vi "Load Words.vi"() -> (3 "Words":string[](array[string]))   [LabVIEW 2020]
uses:
  e4af47f0-1ddf-409f-991e-327bca181c6e.vi
  c56a025f-5e1b-4844-8108-8c9a202df3bb.vi
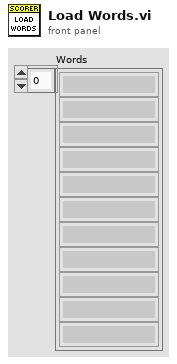
[diagram p1: front panel]
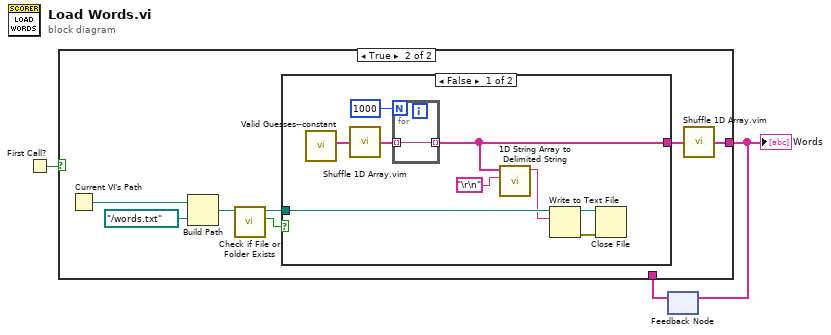
[diagram p0: block diagram]
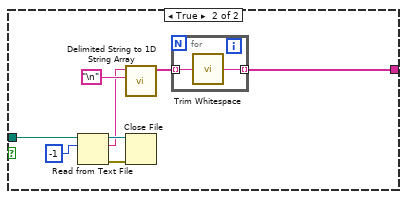
[diagram p3: hidden frame]
diagram:
  n1 = First Call?() -> (First Call?: T/F=w3:bool)
  n2 = feedback #1() -> (w2:string[])  [unwired: 1 in]
  n3 = case shown="True" w3 {
    tunnel: [w4 w6] -> w1
    tunnel: w2 -> [w4 _]
    frame False {
    }
    frame True {
      n4 = Current VI's Path() -> (path=w5:path)
      n5 = Build Path(base path=w5, name or relative path=path "../words.txt") -> (appended path=w10:path)
      n6 = call <vilib>:"Check if File or Folder Exists.vi"("path"=w10) -> ("file or folder exists?"=w9:bool, "dup path"=w8:path)  [unwired: 8 in, 1 out]
      n7 = case shown="False" w9 {
        tunnel: w8 -> [w20 w29]
        tunnel: [w16 w22] -> w7
        frame False {
          n8 = call "Valid Guesses--constant.vi"() -> ("Valid Guesses (array)"=w19:string[])  [unwired: 10 in, 1 out]
          n9 = call "Shuffle 1D Array.vim"("array"=w19) -> ("shuffled array"=w17:string[])  [unwired: 4 in]
          n10 = for {
            N: 1000 -> [_]
            tunnel: w17 -> [w21] mode=indexing
            tunnel: [w21] -> w16 mode=indexing
          }
          n11 = call <vilib>:"1D String Array to Delimited String.vi"("delimiter"="\r\n", "string array"=w16) -> ("delimited string"=w14:string)  [unwired: 9 in]
          n12 = Write to Text File(file (use dialog)=w20, text=w14) -> (refnum out=w13:refnum<file>, error out=w12:errorcluster)  [unwired: 2 in, 1 out]
          n13 = Close File(refnum=w13, error in=w12) -> ()  [unwired: 2 out]
        }
        frame True {
          n14 = Read from Text File(file (use dialog)=w29, count=-1) -> (refnum out=w27:refnum<file>, text=w24:string, error out=w26:errorcluster)  [unwired: 2 in, 1 out]
          n15 = call <vilib>:"Delimited String to 1D String Array.vi"("delimiter"="\n", "delimited string"=w24) -> ("string array"=w23:string[])  [unwired: 9 in]
          n16 = Close File(refnum=w27, error in=w26) -> ()  [unwired: 2 out]
          n17 = for {
            tunnel: w23 -> [w31] mode=indexing
            tunnel: [w30] -> w22 mode=indexing
            n18 = call <vilib>:"Trim Whitespace.vi"("string"=w31) -> ("trimmed string"=w30:string)  [unwired: 1 in]
          }
        }
      }
      n19 = call "Shuffle 1D Array.vim"("array"=w7) -> ("shuffled array"=w6:string[])  [unwired: 4 in]
    }
  }
  "Words" <- w1
  n20 = feedback-in #1(w1) -> ()
